vi "UNSETAGAdll.vi"(8 "error in (no error)":errorcluster) -> (0 "error out":errorcluster)   [LabVIEW 2021]
doc: "subroutine UNSETAGA\n\nLoad original values into arrays changed in the call to SETAGA. This\nroutine resets the values back to those loaded when SETUP was called."
uses:
  REFPROP.dll
panel:
  # "REFPROP-UNSETAGAdll.vi"
  # "void  UNSETAGAdll(void )"
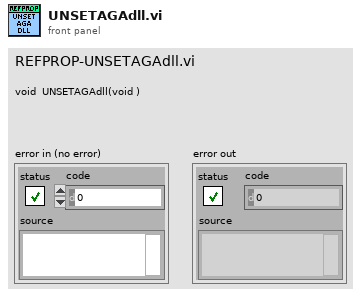
[diagram p1: front panel]
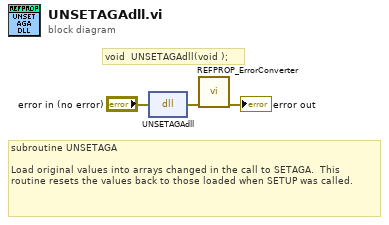
[diagram p0: block diagram]
diagram:
  # "void  UNSETAGAdll(void );"
  # "subroutine UNSETAGA\n\nLoad original values into arrays changed in the call to SETAGA.  This\nroutine resets the values back to those loaded when SETUP was called."
  n1 = dll-call lib="C:/Users/lauria/OneDrive - National Institute of Standards and Technology (NIST)/LabVIEW Projects/7 REFPROP/REFPROP-wrappers-master/REFPROP-wrappers-master/wrappers/Labview/REFPROP/REFPROP.*" fn="UNSETAGAdll"(error in="error in (no error)") -> (error out=w3:errorcluster)  [unwired: 3 in, 1 out]
  n2 = call "REFPROP_ErrorConverter.vi"("error in (no error)"=w3) -> ("error out"=→"error out":errorcluster)  [unwired: 10 in]
